vi "Default Discharge Model.vi"(0 "Rated Capacity (AH)":dbl=100.0, 5 "Discharge Current (A)":dbl=1.0, 7 "Cell Voltage (V)":dbl=3.2, 9 "Cutoff Voltage (V)":dbl=2.8, 11 "Internal Resistance (0.02 Ohm)":dbl=0.02, 12 "Sample Rate (Hz)":i32=1000) -> (6 "Cell Voltage (V)":dbl[](array[numeric]), 8 "Cell Current (A)":dbl[](array[numeric]), 10 "SoC (%)":dbl[](array[numeric]))   [LabVIEW 2023]
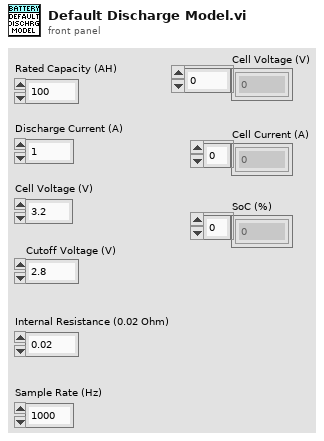
[diagram p1: front panel]
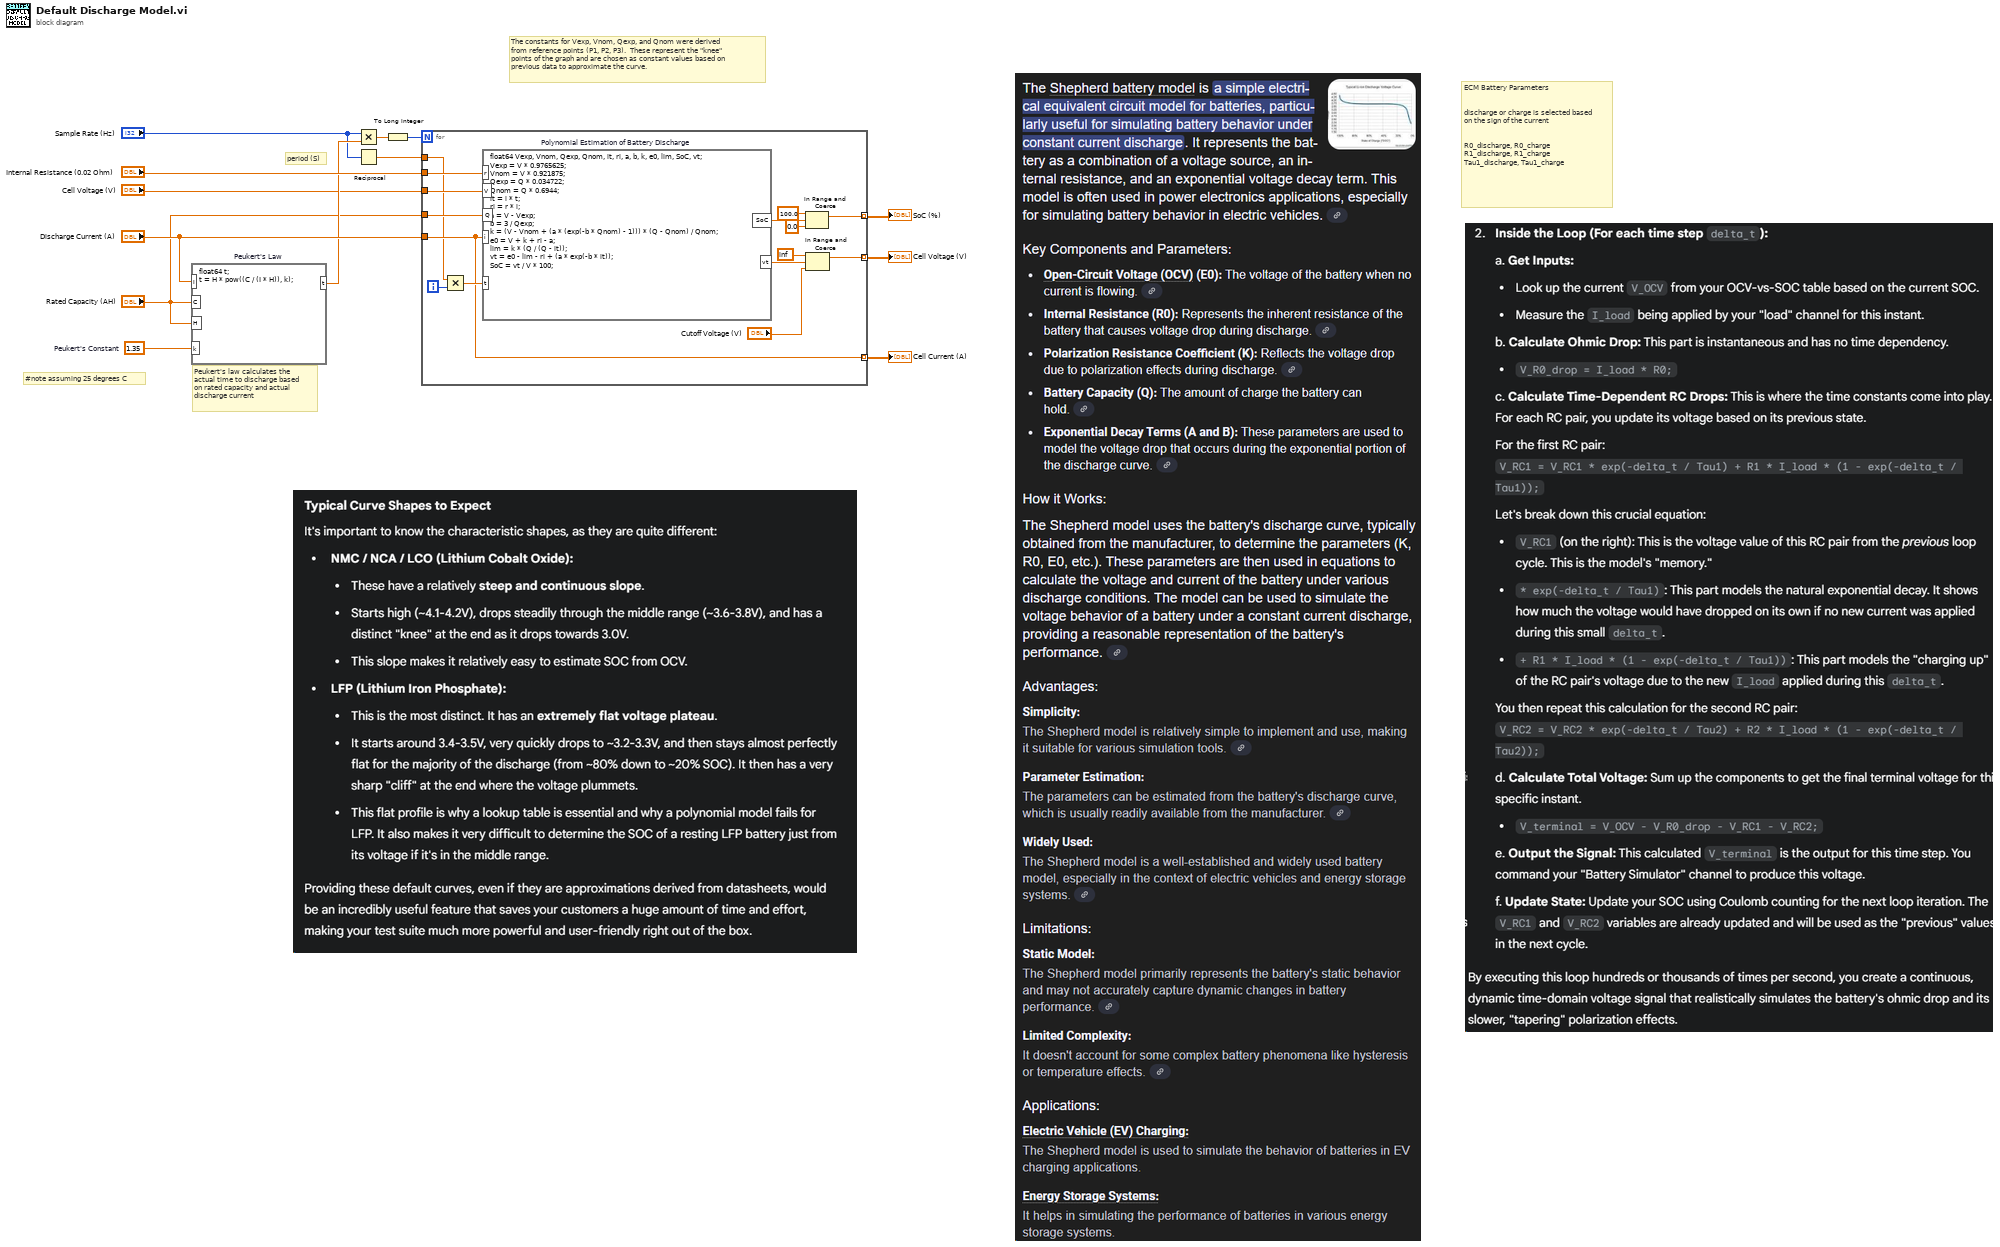
[diagram p0: block diagram]
diagram:
  w10 = 1.35  # Peukert's Constant
  # "ECM Battery Parameters\n\n\ndischarge or charge is selected based\non the sign of the current\n\n\nR0_discharge, R0_charge\nR1_discharge, R1_charge\nTau1_discharge, Tau1_charge"
  # "period (S)"
  # "#note assuming 25 degrees C"
  # "The constants for Vexp, Vnom, Qexp, and Qnom were derived\nfrom reference points (P1, P2, P3).  These represent the \"knee\"\npoints of the graph and are chosen as constant values based on\nprevious data to approximate the curve."
  # "Peukert's law calculates the\nactual time to discharge based\non rated capacity and actual\ndischarge current"
  n1 = formula code="float64 t;\nt = H * pow((C / (I * H)), k);" "Peukert's Law"("k"=w10, "C"="Rated Capacity (AH)", "I"="Discharge Current (A)", "H"="Rated Capacity (AH)") -> ("t"=w11:dbl)
  n2 = Multiply(x="Sample Rate (Hz)", y=w11) -> (x*y=w3:dbl)
  n3 = Reciprocal(x="Sample Rate (Hz)") -> (1/x=w4:dbl)
  n4 = To Long Integer(number=w3) -> (32bit integer=w2:i32)
  n5 = for {
    N: w2 -> [_]
    tunnel: "Cell Voltage (V)" -> [w28]
    tunnel: "Discharge Current (A)" -> [w17]
    tunnel: "Rated Capacity (AH)" -> [w27]
    tunnel: "Internal Resistance (0.02 Ohm)" -> [w26]
    tunnel: [w19] -> w6 mode=indexing
    tunnel: [w18] -> w1 mode=indexing
    tunnel: [w17] -> w7 mode=indexing
    tunnel: w4 -> [w15]
    i -> [w16]
    n6 = Multiply(x=w15, y=w16) -> (x*y=w20:dbl)
    n7 = formula code="float64 Vexp, Vnom, Qexp, Qnom, it, ri, a, b, k, e0, lim, SoC, vt;\nVexp = V * 0.9765625;\nVnom = V * 0.921875;\nQexp = Q * 0.034722;\nQnom = Q * 0.6944;\nit = i * t;\nri = r * i;\na = V - Vexp;\nb = 3 / Qexp;\nk = (V - Vnom + (a * (exp(-b * Qnom) - 1))) * (Q - Qnom) / Qnom;\ne0 = V + k + ri - a;\nlim = k * (Q / (Q - it));\nvt = e0 - lim - ri + (a * exp(-b * it));\nSoC = vt / V * 100;" "Polynomial Estimation of Battery Discharge"("V"=w28, "Q"=w27, "i"=w17, "t"=w20, "r"=w26) -> ("vt"=w25:dbl, "SoC"=w21:dbl)
    n8 = In Range and Coerce(upper limit=100.0, x=w21, lower limit=0.0) -> (coerced(x)=w19:dbl)  [unwired: 1 out]
    n9 = In Range and Coerce(upper limit=inf, x=w25, lower limit="Cutoff Voltage (V)") -> (coerced(x)=w18:dbl)  [unwired: 1 out]
  }
  "Cell Current (A)" <- w7
  "Cell Voltage (V)" <- w1
  "SoC (%)" <- w6
